vi "TDMSAdv writeOfString.vi"(5 "channel name":string, 7 "group name (Untitled)":string, 8 "error in (no error)":errorcluster, 10 "dataArray":string, 11 "TDMSAdv in":refnum<class "TDMSAdv.lvclass">) -> (0 "error out":errorcluster, 3 "TDMSAdv out":refnum<class "TDMSAdv.lvclass">)   [LabVIEW 2018, in "TDMSAdv.lvclass"]
uses:
  TDMSAdv.lvclass
  TDMSAdv.lvclass/TDMSAdv.ctl
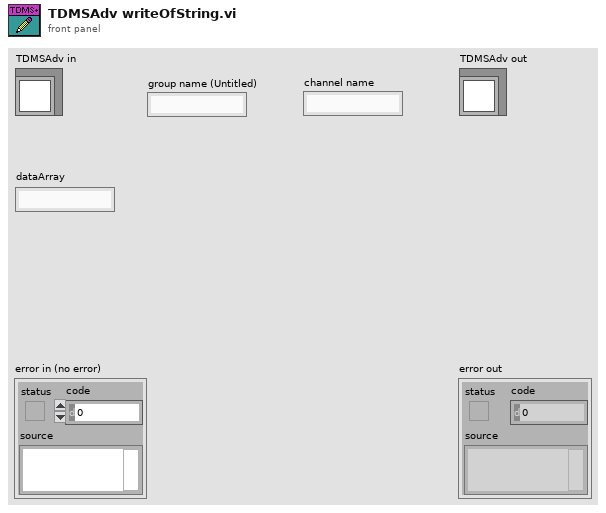
[diagram p1: front panel]
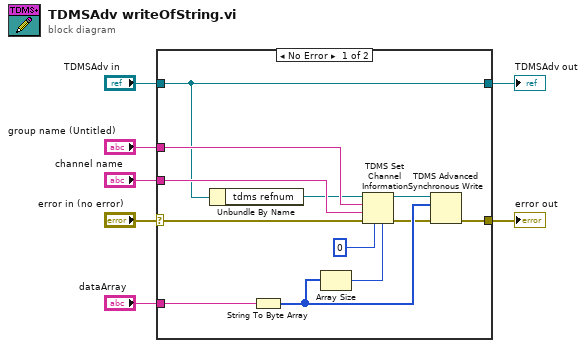
[diagram p0: block diagram]
diagram:
  n1 = case shown="No Error" "error in (no error)" {
    selector: "error in (no error)" -> [w18 w20]
    tunnel: "dataArray" -> [w11 _]
    tunnel: "group name (Untitled)" -> [w17 _]
    tunnel: "channel name" -> [w16 _]
    tunnel: "TDMSAdv in" -> [w14 w21]
    tunnel: [w14 w21] -> w3
    tunnel: [w13 w20] -> w2
    frame No Error {
      n2 = Unbundle By Name(w14) -> ("tdms refnum"=w15:refnum<k34>)
      n3 = String To Byte Array(string=w11) -> (unsigned byte array=w12:u8[])
      n4 = Array Size(array=w12) -> (size(s)=w19:i32)
      n5 = TDMS Set Channel Information(4:w19, 6:u8 0, 8:w18, 9:w16, 10:w17, 11:w15) -> (0:w9:errorcluster, 3:w10:refnum<k34>)  [unwired: 1 in]
      n6 = TDMS Advanced Synchronous Write(8:w9, 10:w12, 11:w10) -> (0:w13:errorcluster)  [unwired: 1 out]
    }
    frame Error {
    }
  }
  "TDMSAdv out" <- w3
  "error out" <- w2
